vi "4-k-dist.vi"(0 "p_LBin":T1, 5 "X=k":i32, 11 "error in (no error)":errorcluster caption="err in") -> (4 "p_LBin":T1, 6 "X=k":i32, 8 "f(X=k)":dbl=0.13261955589475294 caption="f(k) = prob(X=k)", 10 "Fr(X=k)":dbl=0.13261955589475294 caption="F(k) = prob (X<=k)", 15 "error out":errorcluster caption="err out")   [LabVIEW 2010, in "lv_02.lvlib"]
uses:
  p_5E4_LBin.ctl
  <vilib>/gmath/statdist.llb/Binomial CDF.vi
  <vilib>/gmath/statdist.llb/Binomial PF.vi
  lv_02.lvlib
  <vilib>/gmath/NI_Gmath.lvlib
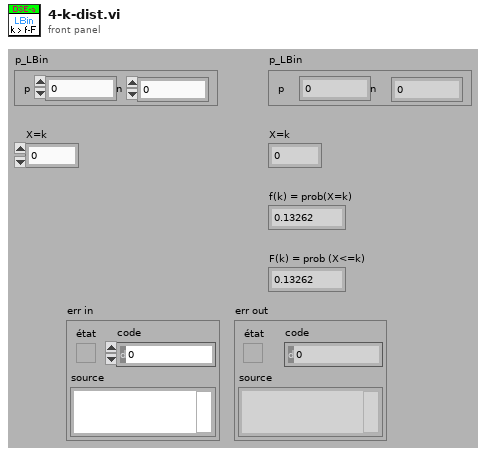
[diagram p1: front panel]
types:
  T1 = typedef "lv_02.lvlib/p_5E4_LBin.ctl" = cluster{"p":dbl, "n":i16}
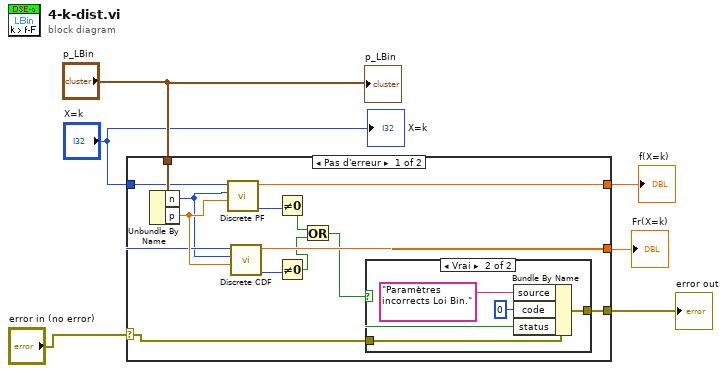
[diagram p0: block diagram]
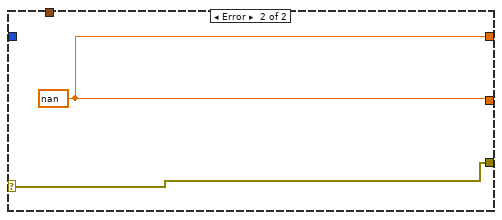
[diagram p3: hidden frame]
diagram:
  n1 = case shown="Pas d'erreur" "error in (no error)" {
    selector: "error in (no error)" -> [w8 w26]
    tunnel: "p_LBin" -> [w19 _]
    tunnel: "X=k" -> [w17 _]
    tunnel: [w15 w27] -> w4
    tunnel: [w14 w27] -> w3
    tunnel: [w7 w26] -> w1
    frame No Error {
      n2 = Unbundle By Name(w19) -> ("n"=w16:i16, "p"=w18:dbl)
      n3 = call-poly <vilib>:"Discrete PF.vi"("p"=w18, "n"=w16, "x"=w17) -> ("error"=w13:i32, "prob(x)"=w15:dbl)  [unwired: 7 in]
      n4 = call-poly <vilib>:"Discrete CDF.vi"("p"=w18, "n"=w16, "x"=w17) -> ("error"=w12:i32, "cdf(x)"=w14:dbl)  [unwired: 7 in]
      n5 = Not Equal To 0?(x=w13) -> (x != 0?=w11:bool)
      n6 = Not Equal To 0?(x=w12) -> (x != 0?=w10:bool)
      n7 = Or(x=w11, y=w10) -> (x .or. y?=w9:bool)
      n8 = case shown="Vrai" w9 {
        selector: w9 -> [_ w24]
        tunnel: w8 -> [w20 w25]
        tunnel: [w20 w21] -> w7
        frame False {
        }
        frame True {
          n9 = Bundle By Name(cluster=w25, "source"="Paramètres incorrects Loi Bin.", "code"=0, "status"=w24) -> (w21:errorcluster)
        }
      }
    }
    frame Error {
      w27 = nan
    }
  }
  "f(X=k)" <- w4
  "Fr(X=k)" <- w3
  "error out" <- w1
  "p_LBin" <- "p_LBin"
  "X=k" <- "X=k"
